vi "Peregrine_set_parameters.vi"(0 "Handle in":refnum<visa-resource-name>, 2 "Address":u8, 7 "Select parameter":T1(ring), 11 "error":errorcluster) -> (4 "Handle out":refnum<visa-resource-name>, 6 "Key response":u32, 10 "Value response":i32, 15 "error out":errorcluster)   [LabVIEW 2019]
panel:
  # "Inputs"
  # "Response message"
  # "Output"
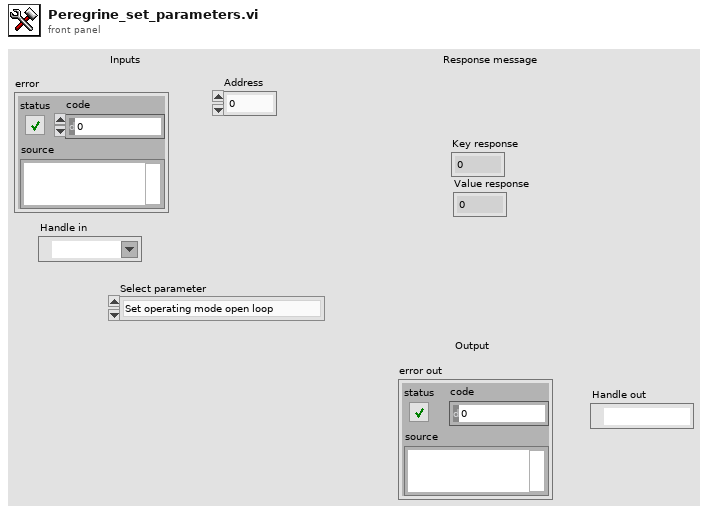
[diagram p1: front panel]
types:
  T1 = enum16{"Set operating mode open loop", "Set operating mode closed loop", "Set path planning OFF", "Set path planning ON", "Set encoder mode to incremental", "Set encoder mode to absolute", "Set encoder mode to absolute multiturn", "Set microstepping to 8", "Set microstepping to 2", "Set microstepping to 4", "Set microstepping to 16", "Limit switch enabled", "Limit switch disabled", "Limit switch inverted", "Control algorithm PID", "Control algorithm LQR", "Power saving mode", "Power always on"}
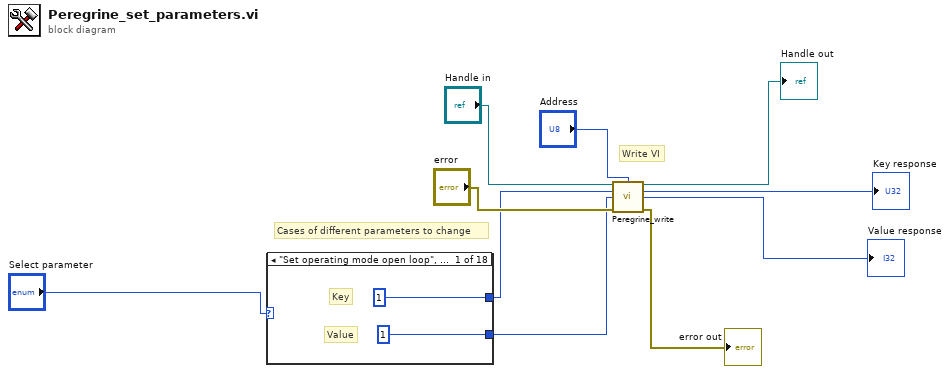
[diagram p0: block diagram]
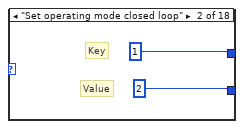
[diagram p2: hidden frame]
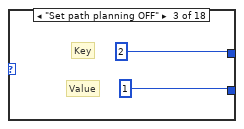
[diagram p3: hidden frame]
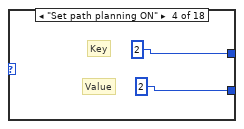
[diagram p4: hidden frame]
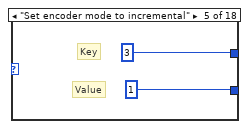
[diagram p5: hidden frame]
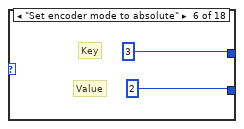
[diagram p6: hidden frame]
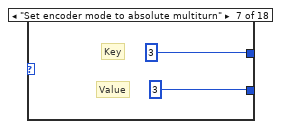
[diagram p7: hidden frame]
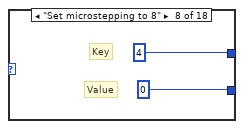
[diagram p8: hidden frame]
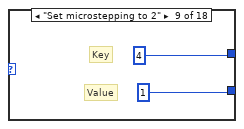
[diagram p9: hidden frame]
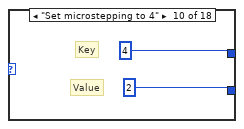
[diagram p10: hidden frame]
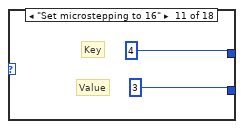
[diagram p11: hidden frame]
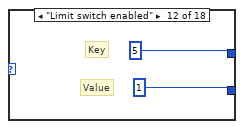
[diagram p12: hidden frame]
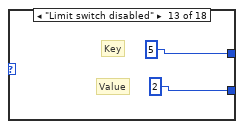
[diagram p13: hidden frame]
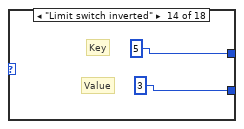
[diagram p14: hidden frame]
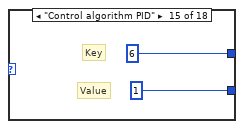
[diagram p15: hidden frame]
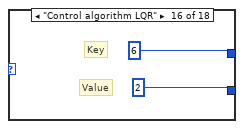
[diagram p16: hidden frame]
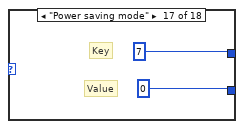
[diagram p17: hidden frame]
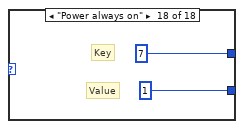
[diagram p18: hidden frame]
diagram:
  # "Cases of different parameters to change"
  # "Write VI"
  n1 = case shown="\"Set operating mode open loop\", Default" "Select parameter" {
    tunnel: [u32 1 u32 1 u32 2 u32 2 u32 3 u32 3 u32 3 u32 4 u32 4 u32 4 u32 4 u32 5 u32 5 u32 5 u32 6 u32 6 u32 7 u32 7] -> w2
    tunnel: [1 2 1 2 1 2 3 0 1 2 3 1 2 3 1 2 0 1] -> w1
    frame "Set operating mode open loop", Default {
      # "Value"
      # "Key"
    }
    frame "Set operating mode closed loop" {
      # "Value"
      # "Key"
    }
    frame "Set path planning OFF" {
      # "Value"
      # "Key"
    }
    frame "Set path planning ON" {
      # "Value"
      # "Key"
    }
    frame "Set encoder mode to incremental" {
      # "Value"
      # "Key"
    }
    frame "Set encoder mode to absolute" {
      # "Value"
      # "Key"
    }
    frame "Set encoder mode to absolute multiturn" {
      # "Value"
      # "Key"
    }
    frame "Set microstepping to 8" {
      # "Value"
      # "Key"
    }
    frame "Set microstepping to 2" {
      # "Value"
      # "Key"
    }
    frame "Set microstepping to 4" {
      # "Value"
      # "Key"
    }
    frame "Set microstepping to 16" {
      # "Value"
      # "Key"
    }
    frame "Limit switch enabled" {
      # "Value"
      # "Key"
    }
    frame "Limit switch disabled" {
      # "Value"
      # "Key"
    }
    frame "Limit switch inverted" {
      # "Value"
      # "Key"
    }
    frame "Control algorithm PID" {
      # "Value"
      # "Key"
    }
    frame "Control algorithm LQR" {
      # "Value"
      # "Key"
    }
    frame "Power saving mode" {
      # "Value"
      # "Key"
    }
    frame "Power always on" {
      # "Value"
      # "Key"
    }
  }
  n2 = call "Peregrine_write.vi"("Handle in"="Handle in", "Address"="Address", "Key"=w2, "Value"=w1, "error"="error") -> ("Handle out"=→"Handle out":refnum<visa-resource-name>, "Key response"=→"Key response":u32, "Value response"=→"Value response":i32, "error out"=→"error out":errorcluster)  [unwired: 7 in]
